vi "飞行姿态模拟.vi"() -> ()   [LabVIEW 2014]
uses:
  <vilib>/picture/3D Picture Control/Object/Create Object (name).vi
  <vilib>/picture/3D Picture Control/Object/Add Object (reference).vi
  <vilib>/Utility/file.llb/Read From Spreadsheet File (DBL).vi
  <vilib>/picture/3D Picture Control/NI_3D Picture Control.lvlib
panel:
  out "三维图片":refnum<vi>(3d-picture)
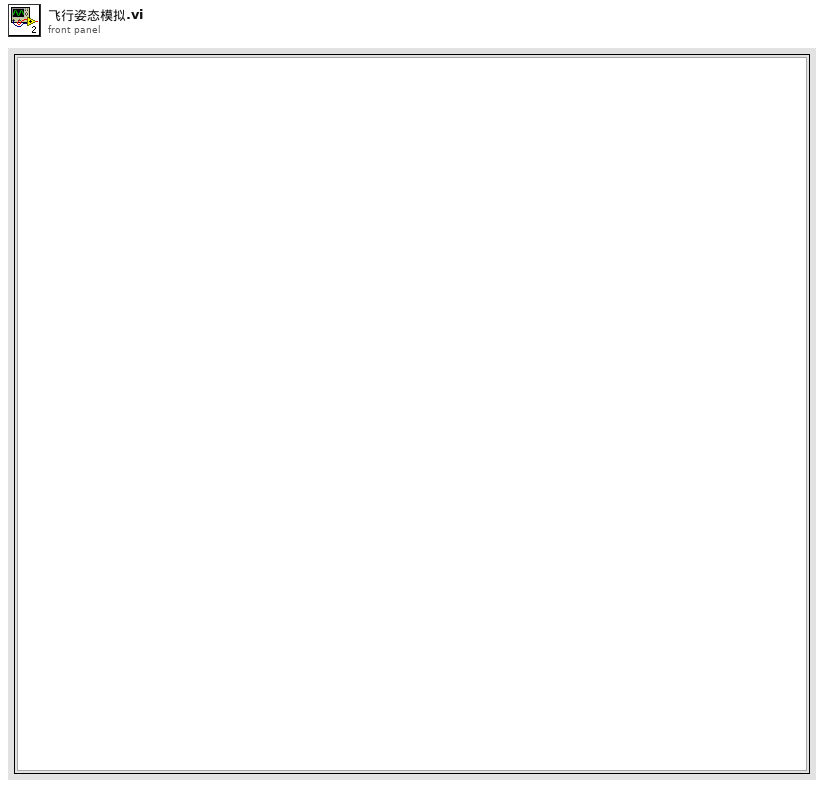
[diagram p1: front panel]
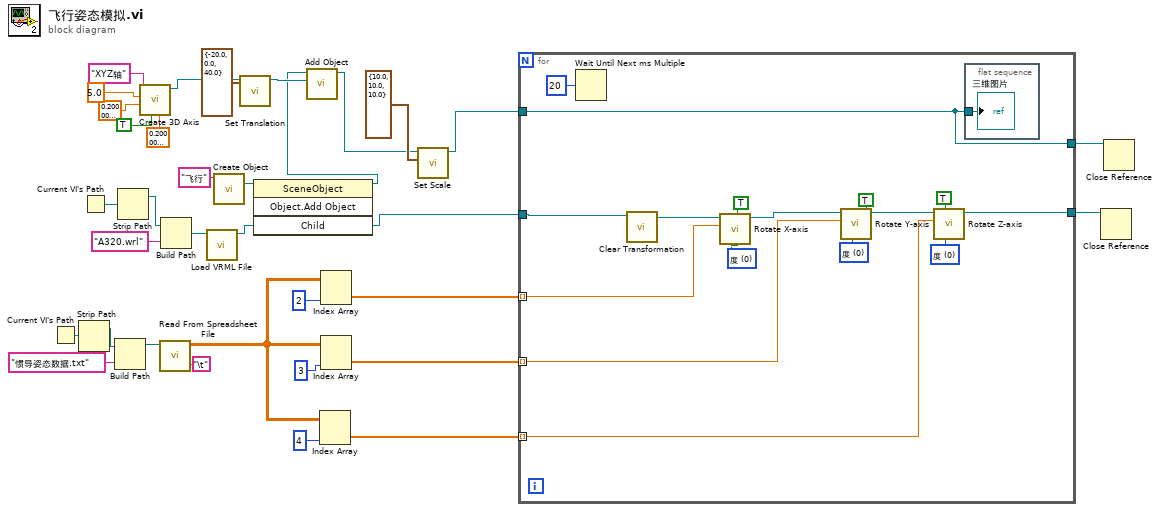
[diagram p0: block diagram]
diagram:
  n1 = Current VI's Path() -> (path=w6:path)
  n2 = Strip Path(path=w6) -> (stripped path=w7:path)  [unwired: 1 out]
  n3 = Current VI's Path() -> (path=w32:path)
  n4 = Build Path(base path=w7, name or relative path="惯导姿态数据.txt" ("名称或相对路径")) -> (appended path=w5:path)
  n5 = Strip Path ("拆分路径")(path=w32) -> (stripped path=w31:path)  [unwired: 1 out]
  n6 = call <vilib>:"Create 3D Axis.vi"("Character Size"=sgl 0.2, "Axis label?"=TRUE, "Radius"=sgl 0.2, "Length"=sgl 5.0, "Name"="XYZ轴") -> ("New Object Refnum"=w17:refnum<vi>)  [unwired: 5 in, 1 out]
  n7 = call-poly <vilib>:"Read From Spreadsheet File.vi"("delimiter (\\t)"="\t" ("delimiter (\\t)"), "file path (dialog if empty)"=w5) -> ("all rows"=w8:dbl[][])  [unwired: 5 in, 4 out]
  n8 = Build Path ("创建路径")(base path=w31, name or relative path="A320.wrl" ("名称或相对路径")) -> (appended path=w29:path)
  n9 = call <vilib>:"Load VRML File.vi"("Path"=w29) -> ("Scene:Read Scene File"=w25:refnum<vi>)  [unwired: 9 in, 1 out]
  n10 = call-poly <vilib>:"Create Object.vi"("Name"="飞行") -> ("Scene:New Object"=w28:refnum<vi>)  [unwired: 9 in, 1 out]
  n11 = call <vilib>:"Set Translation.vi"("Translation"=cluster{"X":sgl, "Y":sgl, "Z":sgl} {"X"=-20.0, "Y"=0.0, "Z"=40.0}, "Scene Object"=w17) -> ("Translated Object"=w16:refnum<vi>)  [unwired: 8 in, 1 out]
  n12 = invoke class="SceneObject" method="Object.Add Object"(reference=w28, "Child"=w25) -> (reference out=w15:refnum<vi>, "Child"=w14:refnum<vi>)  [unwired: 2 in, 2 out]
  n13 = call-poly <vilib>:"Add Object.vi"("New Object In"=w16, "Scene Object In"=w15) -> ("Scene Object Out"=w18:refnum<vi>)  [unwired: 7 in, 2 out]
  n14 = Index Array(array=w8, index (col)=4 ("禁用的索引 (列)")) -> (element=w1:dbl[])  [unwired: 1 in]
  n15 = Index Array(array=w8, index (col)=2 ("禁用的索引 (列)")) -> (element=w3:dbl[])  [unwired: 1 in]
  n16 = Index Array(array=w8, index (col)=3 ("禁用的索引 (列)")) -> (element=w2:dbl[])  [unwired: 1 in]
  n17 = call <vilib>:"Set Scale.vi"("Scale"=cluster{"X":sgl, "Y":sgl, "Z":sgl} {"X"=10.0, "Y"=10.0, "Z"=10.0}, "Scene Object"=w18) -> ("Scaled Object"=w13:refnum<vi>)  [unwired: 8 in, 1 out]
  n18 = for {
    tunnel: w13 -> [w41]
    tunnel: w14 -> [w42]
    tunnel: [w41] -> w34
    tunnel: [w40] -> w33
    tunnel: w3 -> [w36] mode=indexing
    tunnel: w2 -> [w35] mode=indexing
    tunnel: w1 -> [w37] mode=indexing
    w47 = u16 0 items=["度", "弧度"] ("angle unit")
    w48 = u16 0 items=["度", "弧度"] ("angle unit")
    w49 = u16 0 items=["度", "弧度"] ("angle unit")
    n19 = Wait Until Next ms Multiple(millisecond multiple=u32 20 ("毫秒倍数")) -> ()  [unwired: 1 out]
    n20 = call <vilib>:"Clear Transformation.vi"("Object Refnum In"=w42) -> ("Object Refnum Out"=w44:refnum<vi>)  [unwired: 9 in, 1 out]
    n21 = call <vilib>:"Rotate X-axis.vi"("angle unit"=w49, "Relative?"=TRUE, "angle"=w36, "Scene Object In"=w44) -> ("Scene Object Out"=w46:refnum<vi>)  [unwired: 6 in, 1 out]
    n22 = call <vilib>:"Rotate Y-axis.vi"("angle unit"=w48, "Relative?"=TRUE, "angle"=w35, "Scene Object In"=w46) -> ("Scene Object Out"=w45:refnum<vi>)  [unwired: 6 in, 1 out]
    n23 = call <vilib>:"Rotate Z-axis.vi"("angle unit"=w47, "Relative?"=TRUE, "angle"=w37, "Scene Object In"=w45) -> ("Scene Object Out"=w40:refnum<vi>)  [unwired: 6 in, 1 out]
    n24 = flat-sequence {
      tunnel: w41 -> [w51]
      frame #0 {
        "三维图片" <- w51
      }
    }
  }
  n25 = Close Reference(reference=w33) -> ()  [unwired: 1 in, 1 out]
  n26 = Close Reference(reference=w34) -> ()  [unwired: 1 in, 1 out]
